vi "User Message Tester.vi"   [LabVIEW 2021]
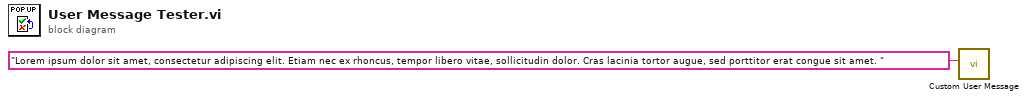
[diagram p0: block diagram]
diagram:
  n1 = call "Custom User Message.vi"("Message"="Lorem ipsum dolor sit amet, consectetur adipiscing elit. Etiam nec ex rhoncus, tempor libero vitae, sollicitudin dolor. Cras lacinia tortor augue, sed porttitor erat congue sit amet. ") -> ()  [unwired: 10 in, 1 out]
